vi "Get Parent ID Priv.vi"(0 "Tree Dictionary":variant, 7 "Unique ID":string, 11 "error in":errorcluster) -> (4 "Tree Dictionary Out":variant, 8 "Parent ID":string, 15 "error out":errorcluster)   [LabVIEW 2016, in "Tree Manager.lvclass"]
uses:
  Tree Manager.lvclass
  Typedefs/Tree.ctl
  <vilib>/Utility/error.llb/Error Cluster From Error Code.vi
  <vilib>/ErrorRing/Error Ring.xnode
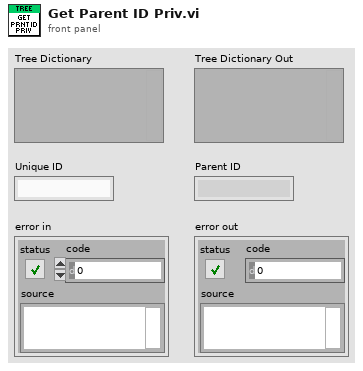
[diagram p1: front panel]
types:
  T1 = typedef "Tree Manager.lvclass/Tree.ctl" = cluster{"Unique ID":string, "Parent ID":string, "Child IDs":string[], "Data":variant, "Name":string}
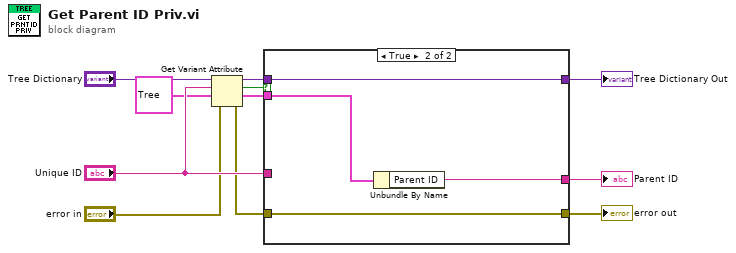
[diagram p0: block diagram]
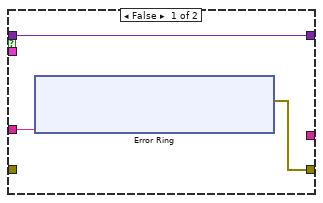
[diagram p2: hidden frame]
diagram:
  n1 = Get Variant Attribute(Variant="Tree Dictionary", name="Unique ID", default value (empty Variant)=T1 {"Unique ID"="", "Parent ID"="", "Child IDs"=[], "Data"=variant, "Name"=""} ("Cluster of class private data"), error in="error in") -> (duplicate Variant=w2:variant, found=w4:bool, value=w3:T1, error out=w1:errorcluster)
  n2 = case shown="True" w4 {
    tunnel: w3 -> [_ w23]
    tunnel: w2 -> [w14 w25]
    tunnel: w1 -> [_ w24]
    tunnel: [w13 w24] -> w9
    tunnel: [w14 w25] -> w7
    tunnel: "Unique ID" -> [w12 _]
    tunnel: [_ w22] -> w11
    frame False {
      n3 = xnode "Error Ring"("parameter 0"=w12) -> ("error out"=w13:errorcluster)
    }
    frame True {
      n4 = Unbundle By Name(w23) -> ("Parent ID"=w22:string)
    }
  }
  "Parent ID" <- w11
  "error out" <- w9
  "Tree Dictionary Out" <- w7
